vi "CPP-BLPowerLawFit.vi"() -> (0 "New Values In":string[][](array[string]), 1 "New Chs In":string[](array[string]))   [LabVIEW 2021]
uses:
  Data plotting/subVIs/Plot_Values_Global.vi
  gnuplotScriptComponents/BLPlottersubVIs/Resampler.ctl
panel:
  in  "Resampler":T1
  in  "ResampleToN":i32=12
  in  "ResampleHeights":dbl[](array[numeric])=[25.4, 38.1, 50.8, 76.2, 101.6, 127.0, 152.4, 203.2, 254.0, 304.8, 406.4, 508.0, 609.6, 812.8, 1219.2, 1524.0]
  in  "Zref":dbl=508.0
  in  "Fit Zmax":dbl=550.0
  in  "Fit Zmin":dbl=80.0
  # "This VI receives \"classic\" transposed plots of U/Uref vs Z, and fits a power law to them over the range specified on this front panel, for the stated Zref- which will be normalised to internally here.\nBest to do some trial runs to establish a sensible fit range, and then batch process profiles which share common fit ranges."
  # "Fit using values at  measurement Z heights"
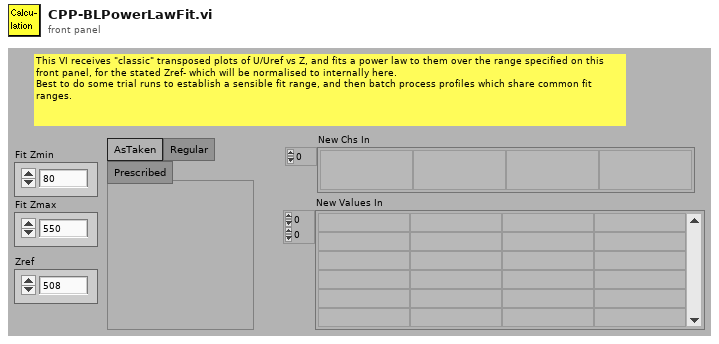
[diagram p1: front panel]
types:
  T1 = typedef "Resampler.ctl" = enum32{"AsTaken", "Regular", "Prescribed"}
  T2 = typedef "PowerLaw.ctl" = cluster{"n":dbl, "d0":dbl, "Residual":dbl}
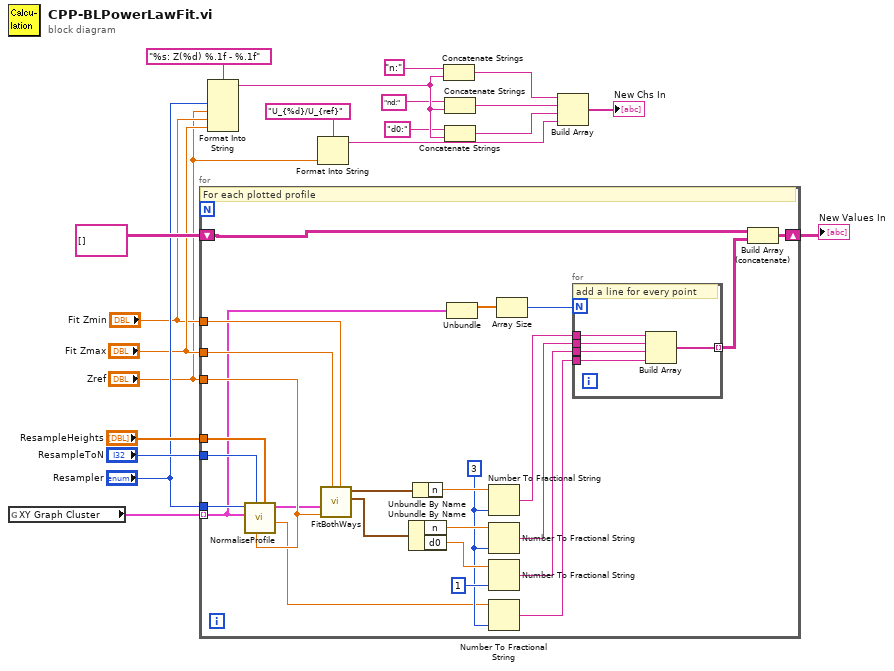
[diagram p0: block diagram]
diagram:
  n1 = global read "Plot_Values_Global.vi" "XY Graph Cluster"() -> (w1:cluster{dbl[], dbl[]}[])
  n2 = for {
    tunnel: "Fit Zmin" -> [w43]
    tunnel: "Fit Zmax" -> [w42]
    tunnel: "Zref" -> [w29]
    tunnel: w1 -> [w24] mode=indexing
    shift-right: [w34] -> w15
    shift-left: string[][] [] -> [w33]
    tunnel: "Resampler" -> [w28]
    tunnel: "ResampleToN" -> [w27]
    tunnel: "ResampleHeights" -> [w26]
    w23 = i16 3 ("precision (6)")
    # "For each plotted profile"
    n3 = call "NormaliseProfile.vi"("ResampleHeights"=w26, "Zref"=w29, "ResampleToN"=w27, "UzClusterIn"=w24, "Resampler"=w28) -> ("U(Zref)"=w22:dbl, "UzClusterOutput"=w25:cluster{dbl[], dbl[]})  [unwired: 5 in]
    n4 = call "FitBothWays.vi"("Fit Zmin"=w43, "Fit Zmax"=w42, "Zref"=w29, "zUCluster in"=w25) -> ("PowerLawWithDisplacement"=w44:T2, "PowerLawNoDisplacement"=w45:T2)  [unwired: 6 in]
    n5 = Unbundle By Name(w44) -> ("n"=w40:dbl, "d0"=w39:dbl)
    n6 = Unbundle By Name(w45) -> ("n"=w41:dbl)
    n7 = Unbundle(w24) -> (w31:dbl[])  [unwired: 1 out]
    n8 = Number To Fractional String(number=w41, precision (6)=w23) -> (F-format string=w37:string)  [unwired: 2 in]
    n9 = Number To Fractional String(number=w40, precision (6)=w23) -> (F-format string=w36:string)  [unwired: 2 in]
    n10 = Number To Fractional String(number=w39, precision (6)=i16 1) -> (F-format string=w35:string)  [unwired: 2 in]
    n11 = Number To Fractional String(number=w22, precision (6)=w23) -> (F-format string=w21:string)  [unwired: 2 in]
    n12 = Array Size(array=w31) -> (size(s)=w32:i32)
    n13 = for {
      N: w32 -> [_]
      tunnel: w37 -> [w50]
      tunnel: w36 -> [w49]
      tunnel: w35 -> [w48]
      tunnel: [w47] -> w30 mode=indexing
      tunnel: w21 -> [w46]
      # "add a line for every point"
      n14 = Build Array(w50, w49, w48, w46) -> (w47:string[])
    }
    n15 = Build Array (concatenate)(w33, w30) -> (w34:string[][])
  }
  "New Values In" <- w15
  n16 = Format Into String(format string="%s: Z(%d) %.1f - %.1f", "Resampler", "Zref", "Fit Zmin", "Fit Zmax") -> (resulting string=w11:string)  [unwired: 2 in, 1 out]
  n17 = Format Into String(format string="U_{%d}/U_{ref}", "Zref") -> (resulting string=w4:string)  [unwired: 2 in, 1 out]
  n18 = Concatenate Strings("n:" ("string"), w11) -> (w19:string)
  n19 = Concatenate Strings("nd:" ("string"), w11) -> (w18:string)
  n20 = Concatenate Strings("d0:" ("string"), w11) -> (w17:string)
  n21 = Build Array(w19, w18, w17, w4) -> (→"New Chs In":string[])
